vi "C(T) Trigger checker.vi"(1 "Raw C(T) data array":dbl[][](array[numeric]) format="%.2f") -> (0 "trigger was correct polarity":bool)   [LabVIEW 2016]
doc: "this subvi checks that the positive edge voltage was triggered on the way up to a high voltage instead of on the way down due to a fluctuation\n\nPaul K Dixon\nPhysics 350\nCSUSB Physics"
uses:
  <vilib>/Analysis/baseanly.llb/Mean (DBL).vi
  <vilib>/Analysis/NI_AALBase.lvlib
panel:
  # "C(T) trigger checker"
  # "baseline"
  # "decay"
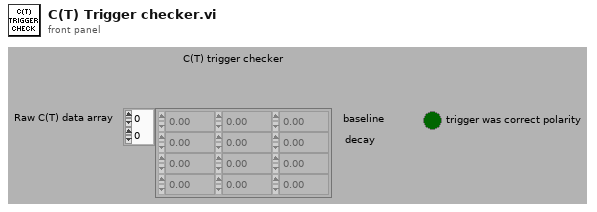
[diagram p1: front panel]
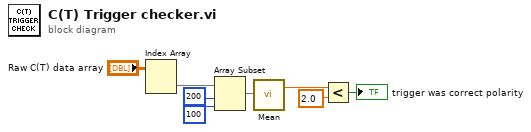
[diagram p0: block diagram]
diagram:
  n1 = Index Array(array="Raw C(T) data array") -> (element=w3:dbl[])  [unwired: 2 in]
  n2 = Array Subset(array=w3, index=200 ("Array Index"), length=100 ("Array Length")) -> (w4:dbl[])
  n3 = call-poly <vilib>:"Mean.vi"("X"=w4) -> ("mean"=w5:dbl)  [unwired: 1 out]
  n4 = Less?(x=w5, y=2.0) -> (x < y?=→"trigger was correct polarity":bool)
